vi "Config Home.vi"(0 "Homing direction invert":T1, 1 "Homing cycle enable":bool, 5 "Homing locate feed rate\tmm/min":u32=25, 7 "Homing search seek rate\tmm/min":u32=255, 9 "Homing switch debounce delay\tms":u32=255, 11 "error in (no error)":errorcluster, 12 "Homing switch pull-off distance\tmm":u32=255) -> (15 "error out":errorcluster)   [LabVIEW 2024, in "GRBL 1.1.lvlib"]
doc: "Homing cycle enable: Enables homing cycle. Requires limit switches on all axes.\nHoming direction invert: Homing searches for a switch in the positive direction. Set axis bit (00000ZYX) to search in negative direction.\nHoming locate feed rate: Feed rate to slowly engage limit switch to determine its location accurately.\nHoming search seek rate: Seek rate to quickly find the limit switch before the slower locating phase.\nHoming switch debounce delay: Sets a short delay between phases of homing cycle to let a switch debounce.\nHoming switch pull-off distance: Retract distance after triggering switch to disengage it. Homing will fail if switch isn't cleared."
uses:
  GRBL 1.1.lvlib
panel:
  out "Data read":string
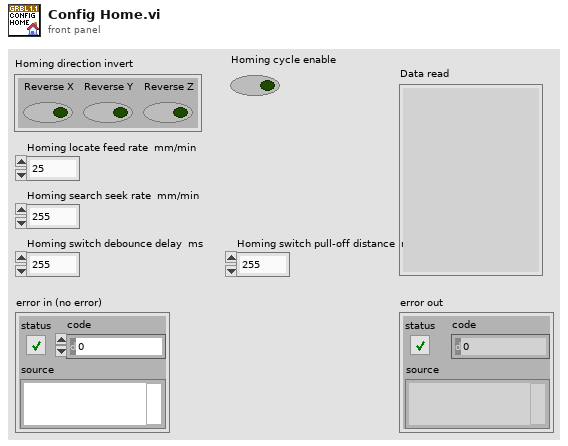
[diagram p1: front panel]
types:
  T1 = cluster{"Reverse X":bool, "Reverse Y":bool, "Reverse Z":bool}
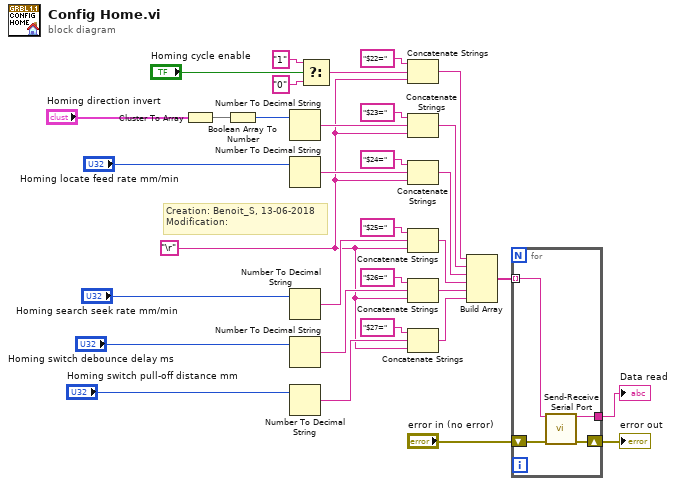
[diagram p0: block diagram]
diagram:
  w8 = "\r"
  # "Creation: Benoit_S, 13-06-2018\nModification:"
  n1 = Cluster To Array(cluster="Homing direction invert") -> (array=w27:bool[])
  n2 = Boolean Array To Number(Boolean array=w27) -> (number=w23:u32)
  n3 = Number To Decimal String(number=w23) -> (decimal integer string=w24:string)  [unwired: 1 in]
  n4 = Number To Decimal String(number="Homing locate feed rate\tmm/min") -> (decimal integer string=w22:string)  [unwired: 1 in]
  n5 = Number To Decimal String(number="Homing search seek rate\tmm/min") -> (decimal integer string=w17:string)  [unwired: 1 in]
  n6 = Number To Decimal String(number="Homing switch debounce delay\tms") -> (decimal integer string=w16:string)  [unwired: 1 in]
  n7 = Number To Decimal String(number="Homing switch pull-off distance\tmm") -> (decimal integer string=w11:string)  [unwired: 1 in]
  n8 = Select(t="1", s="Homing cycle enable", f="0") -> (s? t:f=w30:string)
  n9 = Concatenate Strings("$22=", w30, w8) -> (w7:string)
  n10 = Concatenate Strings("$23=", w24, w8) -> (w6:string)
  n11 = Concatenate Strings("$24=", w22, w8) -> (w5:string)
  n12 = Concatenate Strings("$25=", w17, w8) -> (w4:string)
  n13 = Concatenate Strings("$26=", w16, w8) -> (w3:string)
  n14 = Concatenate Strings("$27=", w11, w8) -> (w2:string)
  n15 = Build Array(w7, w6, w5, w4, w3, w2) -> (w1:string[])
  n16 = for {
    tunnel: [w35] -> w9
    shift-right: [w36] -> w32
    shift-left: "error in (no error)" -> [w37]
    tunnel: w1 -> [w34] mode=indexing
    n17 = call "Send-Receive Serial Port.vi"("Data to write"=w34, "error in (no error)"=w37) -> ("Data read"=w35:string, "error out"=w36:errorcluster)  [unwired: 12 in]
  }
  "error out" <- w32
  "Data read" <- w9
